vi "prompt_fgv.vi"(1 "?":T1, 2 "String in":string) -> (0 "String out":string)   [LabVIEW 2016, in "labssh_thijs.lvlib"]
uses:
  labssh_thijs.lvlib
  store retrieve.ctl
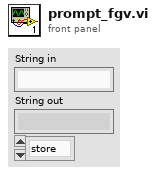
[diagram p1: front panel]
types:
  T1 = typedef "labssh_thijs.lvlib/store retrieve.ctl" = enum16{"store", "retrieve"}
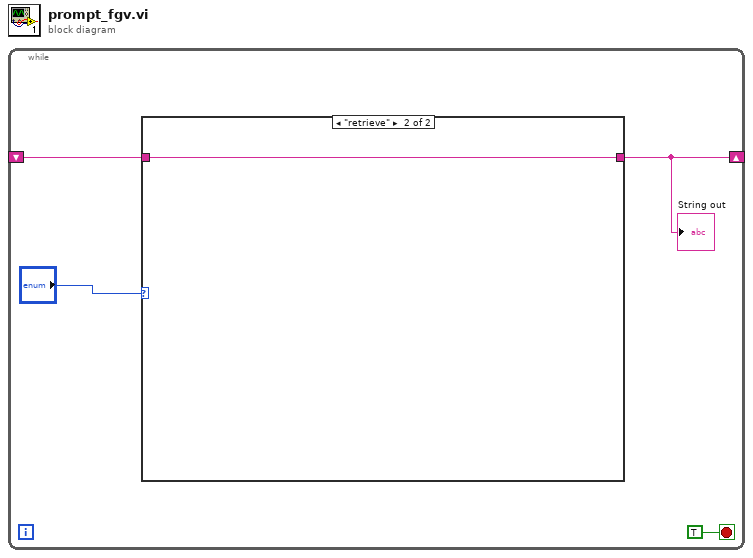
[diagram p0: block diagram]
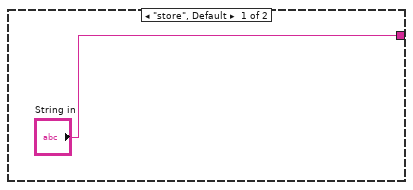
[diagram p2: hidden frame]
diagram:
  n1 = while {
    shift-right: [w2] -> _
    shift-left: _ -> [w3]
    stop <- TRUE stop-if-true
    n2 = case shown="\"retrieve\"" "?" {
      tunnel: ["String in" w6] -> w2
      tunnel: w3 -> [_ w6]
      frame "store", Default {
      }
      frame "retrieve" {
      }
    }
    "String out" <- w2
  }
